vi "getAllUnrestrictedChannels.vi"(8 "error in (no error)":errorcluster, 11 "device in":refnum<class "device.lvclass">) -> (0 "error out":errorcluster, 2 "ChannelArray.lvclass":refnum<class "ChannelArray.lvclass">, 3 "device out":refnum<class "device.lvclass">)   [LabVIEW 2009, in "Tools.lvlib" / "DatabaseHelpers.lvlib" / "device.lvclass"]
uses:
  device.lvclass
  ChannelArray/ChannelArray.lvclass
  Channel/Channel.lvclass
  device.lvclass/device.ctl
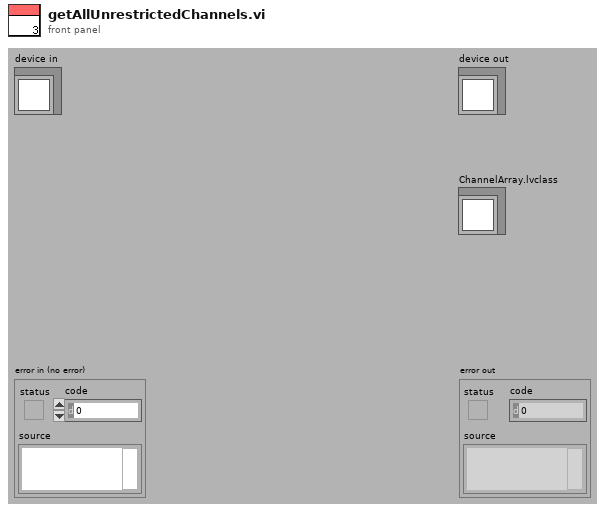
[diagram p1: front panel]
types:
  T1 = cluster{"type":enum16{"restricted", "unrestricted"}, "channel_address":string, "channel_name":string}[]
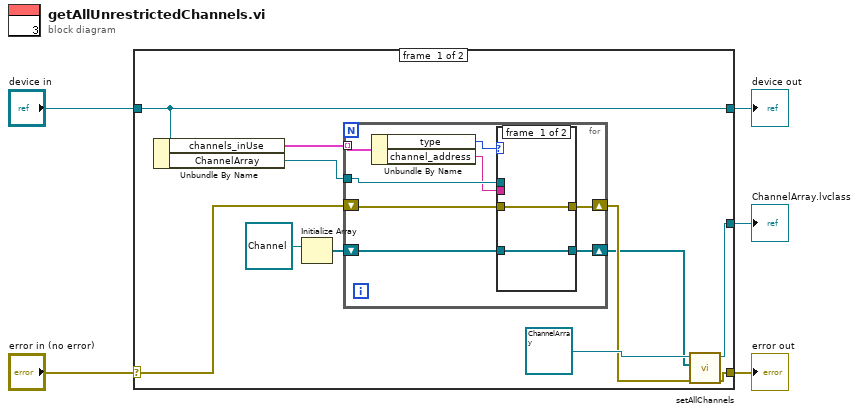
[diagram p0: block diagram]
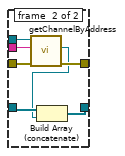
[diagram p2: hidden frame]
diagram:
  n1 = case shown="No Error" "error in (no error)" {
    selector: "error in (no error)" -> [w11 w35]
    tunnel: [w10 w35] -> w4
    tunnel: [w16 w34] -> w2
    tunnel: "device in" -> [w16 w34]
    tunnel: [w9 _] -> w1
    frame #0 {
      n2 = Unbundle By Name(w16) -> ("channels_inUse"=w15:T1, "ChannelArray"=w14:refnum<class "ChannelArray.lvclass">)
      n3 = Initialize Array(refnum<class "Channel.lvclass"> refnum ("Tools.lvlib:DatabaseHelpers.lvlib:Channel.lvclass")) -> (w7:refnum<class "Channel.lvclass">[])  [unwired: 1 in]
      n4 = for {
        tunnel: w15 -> [w24] mode=indexing
        tunnel: w14 -> [w23]
        shift-right: [w20] -> w12
        shift-left: w11 -> [w21]
        shift-right: [w18] -> w6
        shift-left: w7 -> [w17]
        n5 = Unbundle By Name(w24) -> ("type"=w19:enum16{"restricted", "unrestricted"}, "channel_address"=w22:string)
        n6 = case shown="\"unrestricted\"" w19 {
          tunnel: w23 -> [_ w33]
          tunnel: w22 -> [_ w32]
          tunnel: w21 -> [w26 w31]
          tunnel: [w26 w30] -> w20
          tunnel: [w25 w28] -> w18
          tunnel: w17 -> [w25 w29]
          frame #0 {
          }
          frame #1 {
            n7 = call-dynamic "getChannelByAddress.vi"("error in (no error)"=w31, "channel_address"=w32, "ChannelArray in"=w33) -> ("error out"=w30:errorcluster, "Channel"=w27:refnum<class "Channel.lvclass">)  [unwired: 5 in, 2 out]
            n8 = Build Array (concatenate)(w29, w27) -> (w28:refnum<class "Channel.lvclass">[])
          }
        }
      }
      n9 = call "setAllChannels.vi"("error in (no error)"=w12, "channels"=w6, "ChannelArray.lvclass in"=refnum<class "ChannelArray.lvclass"> refnum ("Tools.lvlib:DatabaseHelpers.lvlib:ChannelArray.lvclass")) -> ("error out"=w10:errorcluster, "ChannelArray.lvclass out"=w9:refnum<class "ChannelArray.lvclass">)  [unwired: 7 in]
    }
    frame #1 {
    }
  }
  "error out" <- w4
  "device out" <- w2
  "ChannelArray.lvclass" <- w1
